vi "bh3_data_array_to_data_string.vi"(11 "payload":u8[](array[numeric]) format="%02x") -> (0 "CRC-8":string, 1 "payload":string, 2 "DLC":string, 3 "DLC_payload_CRC":string, 5 "DLC_payload_CRC bytes":u8[](array[numeric]) format="%02x")   [LabVIEW 2013]
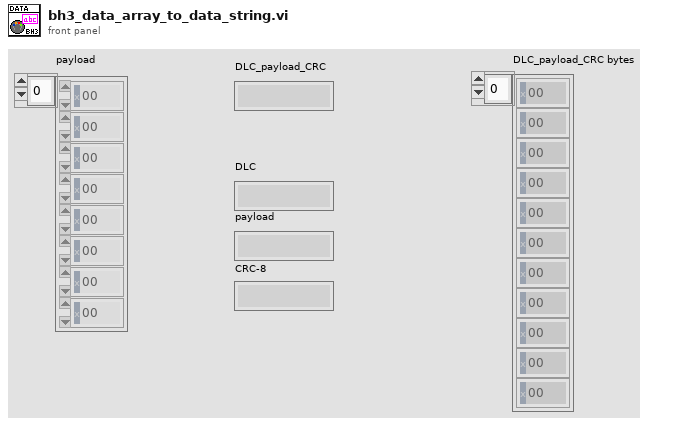
[diagram p1: front panel]
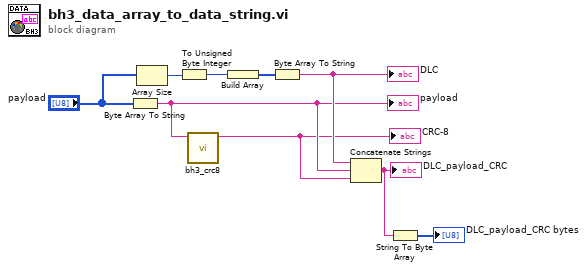
[diagram p0: block diagram]
diagram:
  n1 = Byte Array To String(unsigned byte array="payload") -> (string=w4:string)
  "payload" <- w4
  n2 = Array Size(array="payload") -> (size(s)=w8:i32)
  n3 = To Unsigned Byte Integer(number=w8) -> (unsigned 8bit integer=w7:u8)
  n4 = call "bh3_crc8.vi"("data payload"=w4) -> ("CRC-8 String"=w3:string)  [unwired: 9 in, 1 out]
  "CRC-8" <- w3
  n5 = Build Array(w7) -> (w6:u8[])
  n6 = Byte Array To String(unsigned byte array=w6) -> (string=w5:string)
  "DLC" <- w5
  n7 = Concatenate Strings(w5, w4, w3) -> (w2:string)
  "DLC_payload_CRC" <- w2
  n8 = String To Byte Array(string=w2) -> (unsigned byte array=→"DLC_payload_CRC bytes":u8[])
